vi "Calibrate_temp.vi"(1 "Input":dbl) -> (0 "Output":dbl)   [LabVIEW 2023]
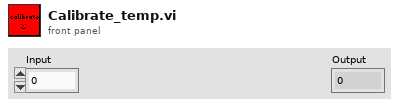
[diagram p1: front panel]
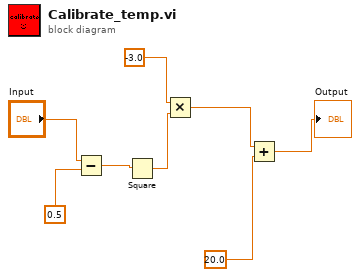
[diagram p0: block diagram]
diagram:
  n1 = Subtract(x="Input", y=0.5) -> (x-y=w6:dbl)
  n2 = Square(x=w6) -> (x^2=w4:dbl)
  n3 = Multiply(x=-3.0, y=w4) -> (x*y=w2:dbl)
  n4 = Add(x=w2, y=20.0) -> (x+y=→"Output":dbl)
